vi "MGCC_StaEst_Testforexe.vi"() -> ()   [LabVIEW 2016]
panel:
  out "standard error 2":string
  out "standard output 2":string
  out "error out":errorcluster
  out "standard error":string
  out "standard output":string
  in  "command line":string
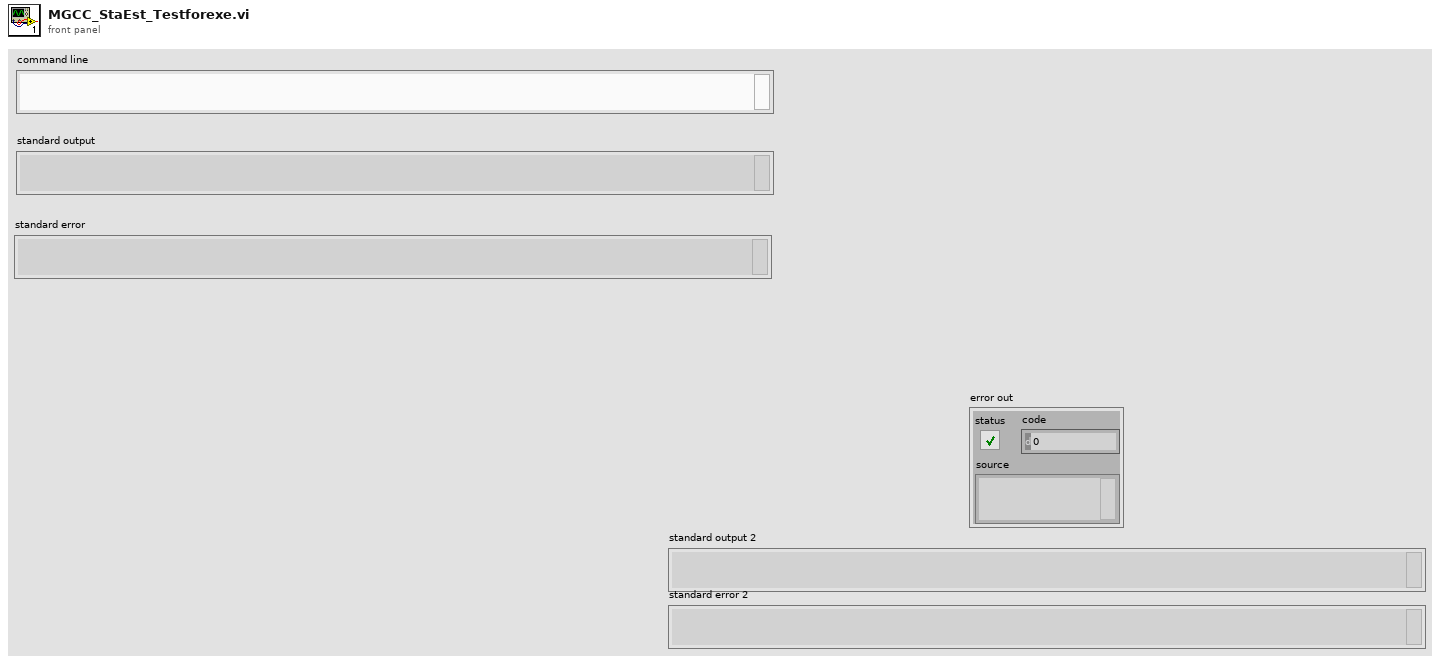
[diagram p1: front panel]
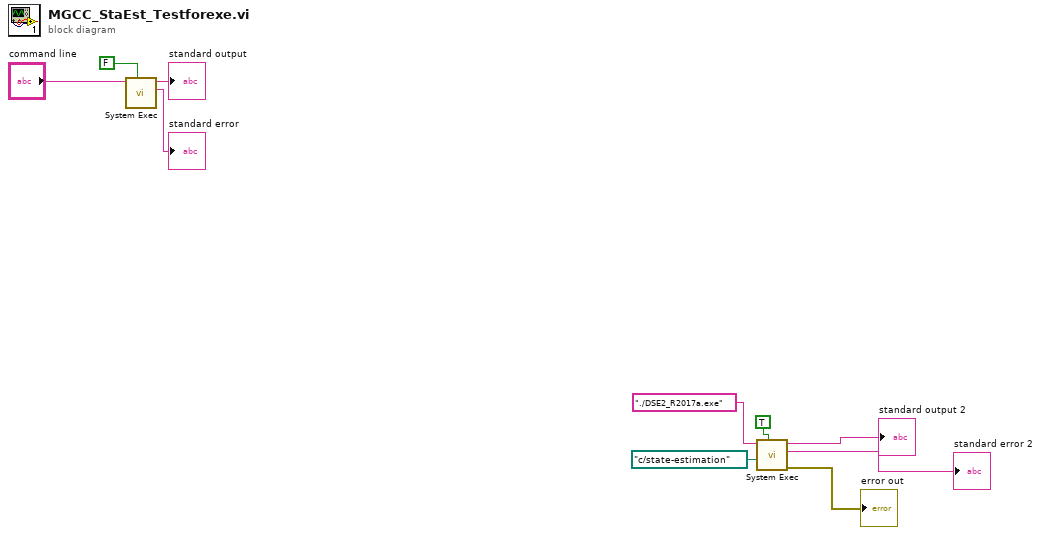
[diagram p0: block diagram]
diagram:
  n1 = call <vilib>:"System Exec.vi"("wait until completion? (T)"=FALSE, "command line"="command line") -> ("standard error"=→"standard error":string, "standard output"=→"standard output":string)  [unwired: 6 in, 2 out]
  n2 = call <vilib>:"System Exec.vi"("wait until completion? (T)"=TRUE ("Wait until done"), "working directory"=path "c:/state-estimation", "command line"="./DSE2_R2017a.exe" ("format string")) -> ("error out"=→"error out":errorcluster, "standard error"=→"standard error 2":string, "standard output"=→"standard output 2":string)  [unwired: 5 in, 1 out]
